vi "SWERVE_SIM_MODULE_MOTOR_OUT.vi"(8 "SwerveOutput":dbl, 9 "DriveOutput":dbl, 10 "SwerveSwerveMotor":T1, 11 "SwervDriveMotor":T1) -> (2 "SwerveMotorDmd":dbl, 3 "WheelMotorDmd":dbl)   [LabVIEW 2019]
uses:
  <vilib>/Rock Robotics/WPI/MotorControl/WPI_MotorControlDeviceRef.ctl
  <vilib>/Rock Robotics/WPI/MotorControl/WPI_MotorControlType.ctl
  <vilib>/Rock Robotics/SystemInterfaces/DIO/FPGA_DIOPWMChannel.ctl
  <vilib>/Rock Robotics/WPI/PWM/WPI_PWMDeadband.ctl
  <vilib>/Rock Robotics/SystemInterfaces/DIO/FPGA_DIOChannel.ctl
  SWERVE_SIM_MODULE_MOTOR_CO.ctl
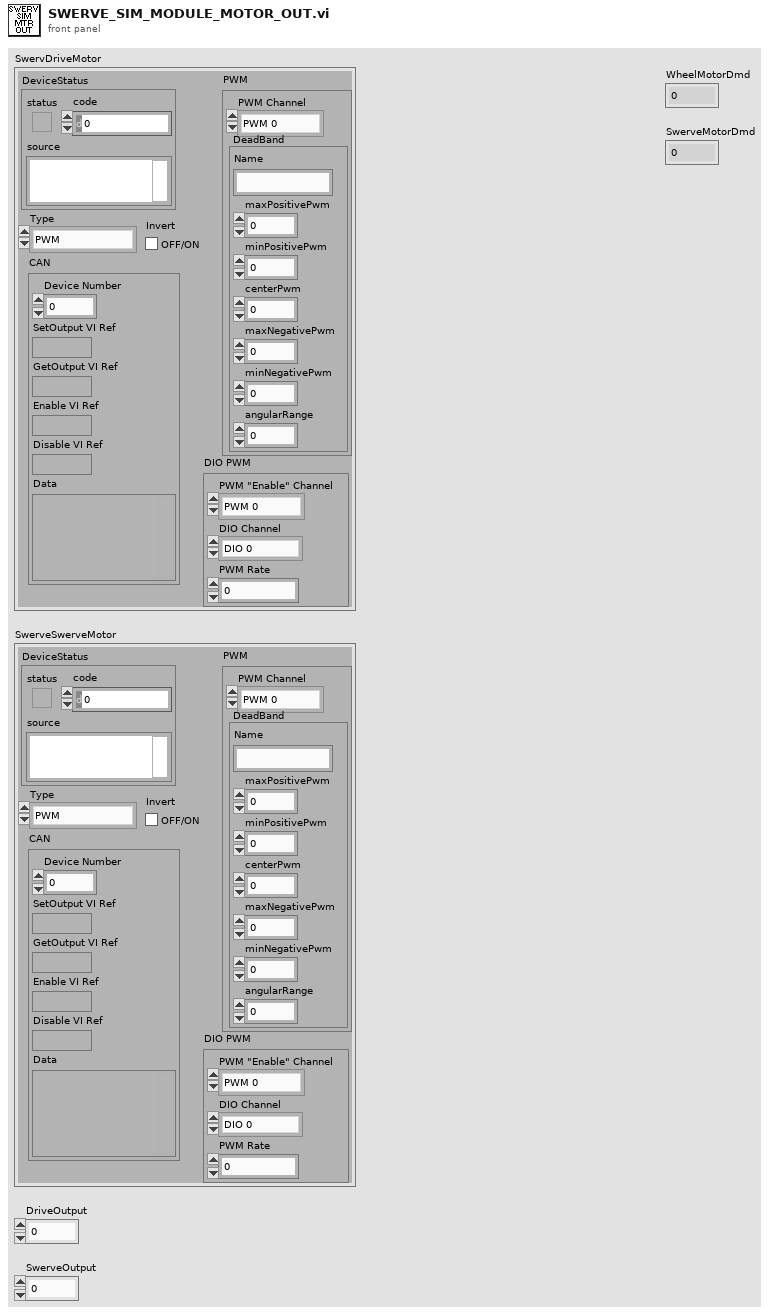
[diagram p1: front panel]
types:
  T1 = typedef "WPI_MotorControlDeviceRef.ctl" = cluster{"DeviceStatus":errorcluster, "Type":T2, "PWM":cluster{"PWM Channel":T3, "DeadBand":T4}, "CAN":cluster{"Device Number":u8, "SetOutput VI Ref":variant, "GetOutput VI Ref":variant, "Enable VI Ref":variant, "Disable VI Ref":variant, "Data":variant}, "Invert":bool, "DIO PWM":cluster{"PWM \"Enable\" Channel":T3, "DIOChannel":T5, "PWM Rate":dbl}}
  T2 = typedef "WPI_MotorControlType.ctl" = enum16{"PWM", "CAN", "DIO PWM"}
  T3 = typedef "FPGA_DIOPWMChannel.ctl" = enum8{"PWM 0", "PWM 1", "PWM 2", "PWM 3", "PWM 4", "PWM 5", "PWM 6", "PWM 7", "PWM 8", "PWM 9", "PWM MXP 0", "PWM MXP 1", "PWM MXP 2", "PWM MXP 3", "PWM MXP 4", "PWM MXP 5", "PWM MXP 6", "PWM MXP 7", "PWM MXP 8", "PWM MXP 9", "Invalid"}
  T4 = typedef "WPI_PWMDeadband.ctl" = cluster{"Name":string, "maxPositivePwm":i32, "minPositivePwm":i32, "centerPwm":i32, "maxNegativePwm":i32, "minNegativePwm":i32, "angularRange":u16}
  T5 = typedef "FPGA_DIOChannel.ctl" = enum8{"DIO 0", "DIO 1", "DIO 2", "DIO 3", "DIO 4", "DIO 5", "DIO 6", "DIO 7", "DIO 8", "DIO 9", "DIO MXP 0", "DIO MXP 1", "DIO MXP 2", "DIO MXP 3", "DIO MXP 4", "DIO MXP 5", "DIO MXP 6", "DIO MXP 7", "DIO MXP 8", "DIO MXP 9", "DIO MXP 10", "DIO MXP 11", "DIO MXP 12", "DIO MXP 13", "DIO MXP 14", "DIO MXP 15", "SPI Port CS1", "SPI Port CS2", "SPI Port CS3", "SPI Port MISO", "SPI Port MOSI", "Invalid"}
  T6 = typedef "SWERVE_SIM_MODULE_MOTOR_CO.ctl" = cluster{"WheelMotorDmd":dbl, "SwerveMotorDmd":dbl}
  T7 = typedef "SWERVE_MODULE_MOTOR_CO.ctl" = cluster{"WheelMotorDmd":dbl, "SwerveMotorDmd":dbl}
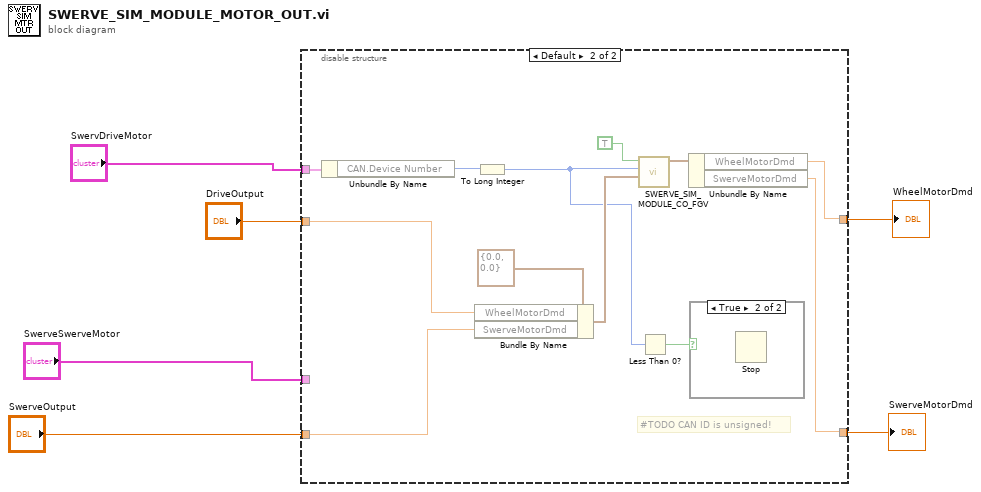
[diagram p0: block diagram]
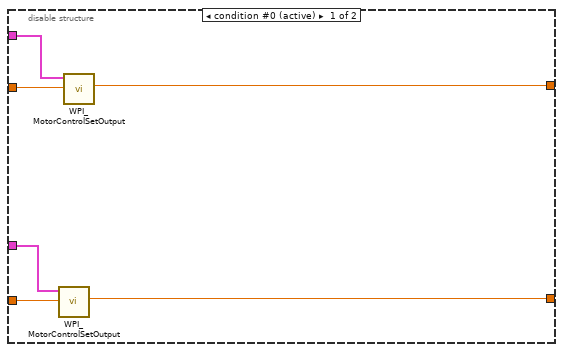
[diagram p2: hidden frame]
diagram:
  n1 = disable-structure shown="Default" {
    disable-tunnel: "SwerveOutput" -> [w12 w20]
    disable-tunnel: "SwerveSwerveMotor" -> [w11 _]
    disable-tunnel: "DriveOutput" -> [w10 w21]
    disable-tunnel: "SwervDriveMotor" -> [w9 w24]
    disable-tunnel: [w8 w16] -> w5
    disable-tunnel: [w7 w15] -> w6
    frame condition #0 (active) {
      n2 = call <vilib>:"WPI_MotorControlSetOutput.vi"("Output"=w12, "MotorControlDevRef"=w11) -> ("Motor Output"=w7:dbl)  [unwired: 7 in, 2 out]
      n3 = call <vilib>:"WPI_MotorControlSetOutput.vi"("Output"=w10, "MotorControlDevRef"=w9) -> ("Motor Output"=w8:dbl)  [unwired: 7 in, 2 out]
    }
    frame condition #1 {
      # "#TODO CAN ID is unsigned!"
      n4 = Unbundle By Name(w24) -> ("CAN.Device Number"=w14:u8)
      n5 = Bundle By Name(cluster=T6 {"WheelMotorDmd"=0.0, "SwerveMotorDmd"=0.0} ("SwerveModuleMotorDmd"), "WheelMotorDmd"=w21, "SwerveMotorDmd"=w20) -> (w19:T6)
      n6 = To Long Integer(number=w14) -> (32bit integer=w13:i32)
      n7 = call "SWERVE_SIM_MODULE_CO_FGV.vi"("in SwerveModuleMotorDmd"=w19, "Index"=w13, "WRITE"=TRUE) -> ("out SwerveModuleMotorDmd"=w17:T7)  [unwired: 8 in]
      n8 = Less Than 0?(x=w13) -> (x < 0?=w18:bool)
      n9 = Unbundle By Name(w17) -> ("WheelMotorDmd"=w16:dbl, "SwerveMotorDmd"=w15:dbl)
      n10 = case shown="True" w18 {
        frame False {
        }
        frame True {
          n11 = Stop() -> ()  [unwired: 1 in]
        }
      }
    }
  }
  "SwerveMotorDmd" <- w6
  "WheelMotorDmd" <- w5
